vi "GetOwningNode.vi"(6 "error in":errorcluster, 9 "ControlTerminal in":refnum<class "ControlTerminal.lvclass">) -> (0 "error out":errorcluster, 3 "ControlTerminal out":refnum<class "ControlTerminal.lvclass">, 4 "node UID":i32)   [LabVIEW 2014, in "ControlTerminal.lvclass"]
uses:
  ControlTerminal.lvclass
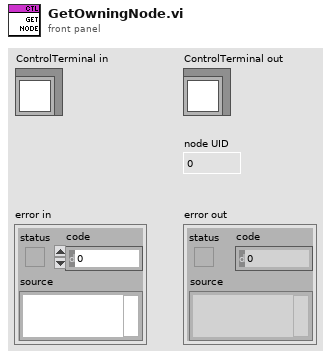
[diagram p1: front panel]
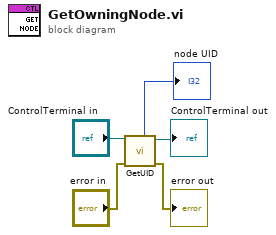
[diagram p0: block diagram]
diagram:
  n1 = call-dynamic "GetUID.vi"("error in"="error in", "GObject in"="ControlTerminal in") -> ("error out"=→"error out":errorcluster, "GObject out"=→"ControlTerminal out":refnum<class "ControlTerminal.lvclass">, "UID"=→"node UID":i32)  [unwired: 5 in]
